vi "Page_Advanced_WriteAll.vi"(6 "ctl references":T1, 8 "error in (no error)":errorcluster, 11 "AB_EXE in":refnum<class "AB_EXE.lvclass">) -> (0 "error out":errorcluster, 3 "AB_EXE out":refnum<class "AB_EXE.lvclass">)   [LabVIEW 2020, in "AB_EXE.lvclass"]
uses:
  <vilib>/AppBuilder/AB_Classes/EXE/AB_EXE.lvclass
  e:/builds/penguin/labview/branches/2020/dev/dist/vi.lib/AppBuilder/AB_Classes/TargetFile/AB_Targetfile.lvclass
  <resource>/Framework/Providers/Builds/AppBuilder/AB_UI_Page_Advanced_References.ctl
  <vilib>/AppBuilder/AB_Classes/EXE/AB_EXE.lvclass/AB_EXE.ctl
  <vilib>/AppBuilder/AB_Classes/Application/AB_Application.lvclass
  <vilib>/AppBuilder/AB_Classes/TargetFile/AB_Targetfile.lvclass
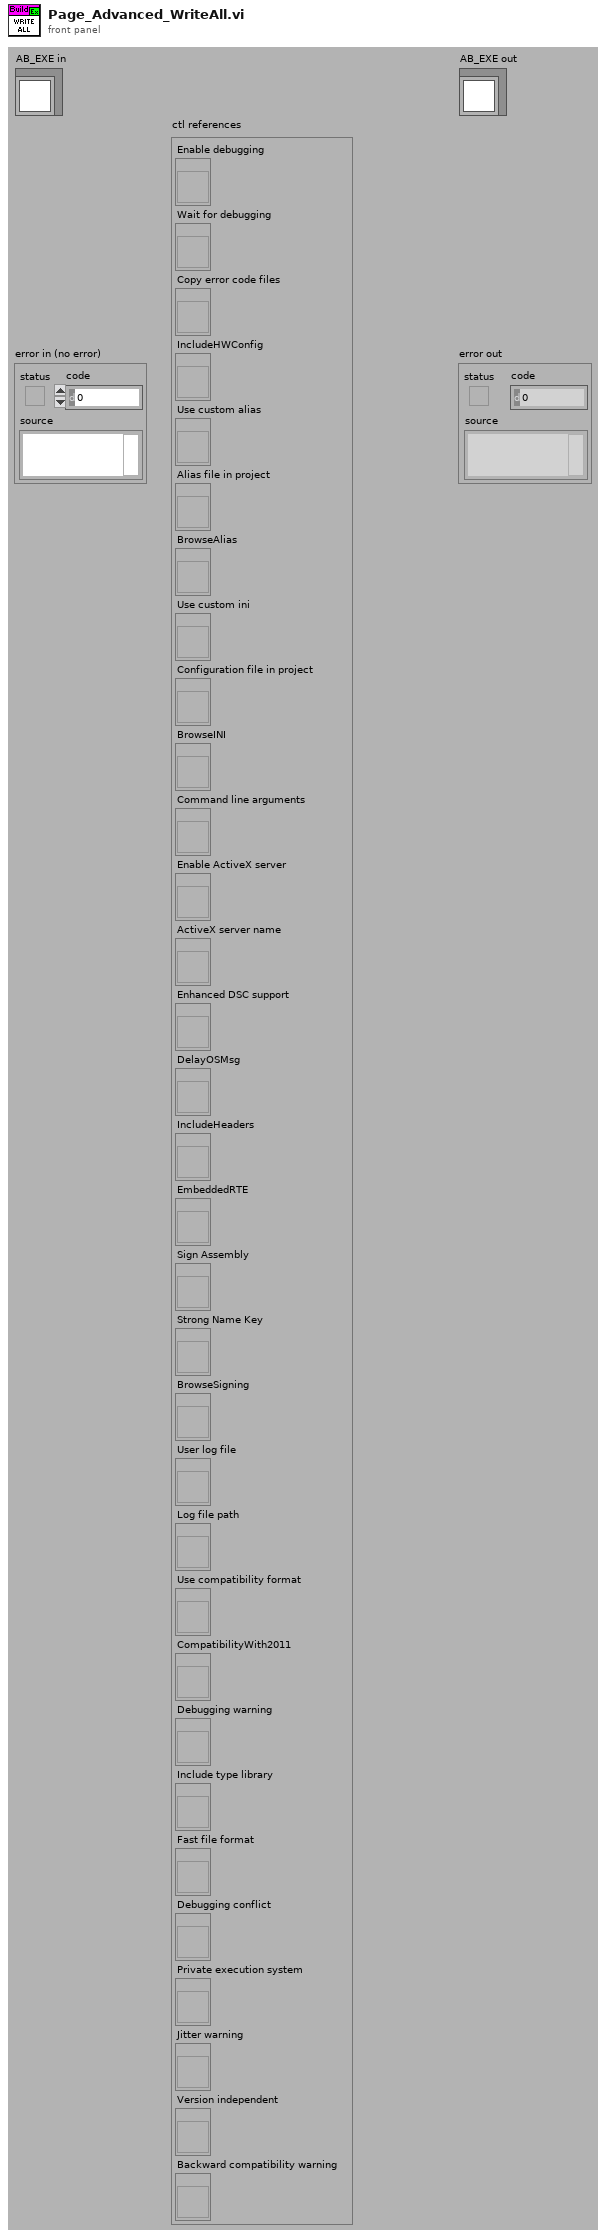
[diagram p1: front panel]
types:
  T1 = typedef "AB_UI_Page_Advanced_References.ctl" = cluster{"Enable debugging":refnum<vi>, "Wait for debugging":refnum<vi>, "Copy error code files":refnum<vi>, "IncludeHWConfig":refnum<vi>, "Use custom alias":refnum<vi>, "Alias file in project":refnum<vi>, "BrowseAlias":refnum<vi>, "Use custom ini":refnum<vi>, "Configuration file in project":refnum<vi>, "BrowseINI":refnum<vi>, "Command line arguments":refnum<vi>, "Enable ActiveX server":refnum<vi>, "ActiveX server name":refnum<vi>, "Enhanced DSC support":refnum<vi>, "DelayOSMsg":refnum<vi>, "IncludeHeaders":refnum<vi>, "EmbeddedRTE":refnum<vi>, "Sign Assembly":refnum<vi>, "Strong Name Key":refnum<vi>, "BrowseSigning":refnum<vi>, "User log file":refnum<vi>, "Log file path":refnum<vi>, "Use compatibility format":refnum<vi>, "CompatibilityWith2011":refnum<vi>, "Debugging warning":refnum<vi>, "Include type library":refnum<vi>, "Fast file format":refnum<vi>, "Debugging conflict":refnum<vi>, "Private execution system":refnum<vi>, "Jitter warning":refnum<vi>, "Version independent":refnum<vi>, "Backward compatibility warning":refnum<vi>}
  T2 = typedef "AB_Targetfile.ctl" = cluster{"targetfileName":string, "targetfileGUID":string, "enableDebugging":bool, "versionInfo":cluster{"productName":string, "legalCopyright":string, "companyName":string, "internalName":string, "fileDescription":string}, "eng_consolidatedTypeInfo":string, "fastFileFormat":bool, "eng_LEIFBuildData":u32, "versionIndependent":bool}
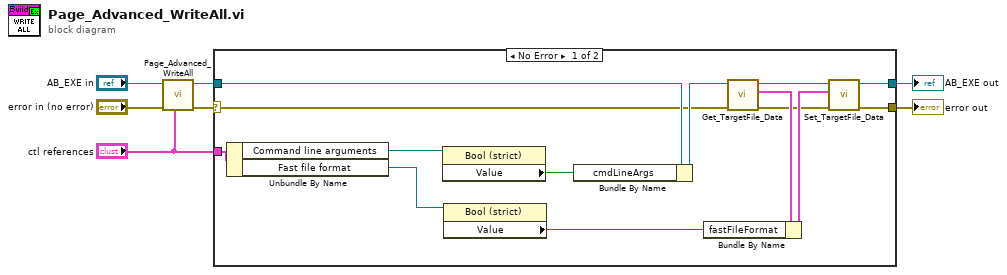
[diagram p0: block diagram]
diagram:
  n1 = call-parent "Page_Advanced_WriteAll.vi"("ctl references"="ctl references", "error in (no error)"="error in (no error)", "AB_Application in"="AB_EXE in") -> ("error out"=w4:errorcluster, "AB_Application out"=w5:refnum<class "AB_EXE.lvclass">)  [unwired: 7 out]
  n2 = case shown="No Error" w4 {
    selector: w4 -> [w10 w22]
    tunnel: w5 -> [w21 w23]
    tunnel: [w11 w23] -> w3
    tunnel: [w8 w22] -> w2
    tunnel: "ctl references" -> [w20 _]
    frame No Error {
      n3 = Unbundle By Name(w20) -> ("Command line arguments"=w19:refnum<vi>, "Fast file format"=w17:refnum<vi>)
      n4 = property class="Bool (strict)"(reference=w19) -> ("Value"=w18:bool)  [unwired: 1 in, 2 out]
      n5 = property class="Bool (strict)"(reference=w17) -> ("Value"=w13:bool)  [unwired: 1 in, 2 out]
      n6 = Bundle By Name(cluster=w21, "cmdLineArgs"=w18) -> (w12:refnum<class "AB_EXE.lvclass">)
      n7 = call <vilib>:"Get_TargetFile_Data.vi"("error in (no error)"=w10, "AB_Targetfile in"=w12) -> ("error out"=w9:errorcluster, "data"=w15:T2, "AB_Targetfile out"=w16:refnum<class "AB_EXE.lvclass">)  [unwired: 7 in]
      n8 = Bundle By Name(cluster=w15, "fastFileFormat"=w13) -> (w14:T2)
      n9 = call <vilib>:"Set_TargetFile_Data.vi"("error in (no error)"=w9, "data"=w14, "AB_Targetfile in"=w16) -> ("error out"=w8:errorcluster, "AB_Targetfile out"=w11:refnum<class "AB_EXE.lvclass">)  [unwired: 7 in]
    }
    frame Error {
    }
  }
  "error out" <- w2
  "AB_EXE out" <- w3
